vi "zero steering.vi"(9 "Power (100)":i8=100, 11 "NXT":T1={"error"={"status"=FALSE, "code"=0, "source"=""}, "address"="", "NXT #"=-1, "Show Error"=TRUE, "Connection"=4} {"Connection" items=["USB", "Bluetooth", "USB then Bluetooth", "Last Connection", "Preference"]}) -> (3 "NXT":T1={"error"={"status"=FALSE, "code"=0, "source"=""}, "address"="", "NXT #"=-1, "Show Error"=TRUE, "Connection"=4} {"Connection" items=["USB", "Bluetooth", "USB then Bluetooth", "Last Connection", "Preference"]})   [LabVIEW 2009]
uses:
  <vilib>/NXT/Subs/LVHSConnector.ctl
  <vilib>/NXT/Subs/MotorOutput.ctl
  <vilib>/NXT/Dual Mode Library/Motors/ResetMotor.vi
  <vilib>/NXT/Dual Mode Library/Motors/MotorBrake.vi
  <vilib>/NXT/Dual Mode Library/Motors/MotorOn.vi
  <vilib>/NXT/Dual Mode Library/Motors/Rotation.vi
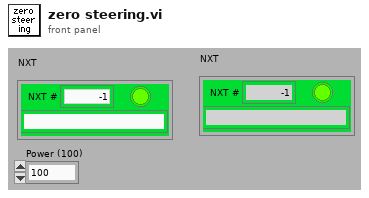
[diagram p1: front panel]
types:
  T1 = typedef "LVHSConnector.ctl" = cluster{"error":errorcluster, "address":string, "NXT #":i32, "Show Error":bool, "Connection":u16}
  T2 = typedef "MotorOutput.ctl" = u8
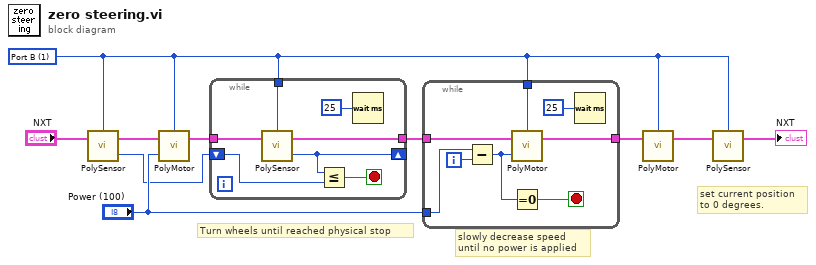
[diagram p0: block diagram]
diagram:
  w3 = T2 1 items=["Port A", "Port B", "Port C", "All Ports"] ("Output Port (All Ports)")
  # "Turn wheels until reached physical stop"
  # "set current position\nto 0 degrees."
  # "slowly decrease speed\nuntil no power is applied"
  n1 = call-poly <vilib>:"PolySensor.vi"("NXT"="NXT", "Port (Port A)"=w3) -> ("Rotation"=w1:i32, "NXT"=w4:T1)  [unwired: 1 in]
  n2 = call-poly <vilib>:"PolyMotor.vi"("Power (75)"="Power (100)", "NXT"=w4, "Output Port (All Ports)"=w3) -> ("NXT"=w2:T1)  [unwired: 1 in]
  n3 = while {
    tunnel: w2 -> [w16]
    tunnel: w3 -> [w17]
    tunnel: [w15] -> w6
    shift-right: [w13] -> _
    shift-left: w1 -> [w12]
    stop <- w11 stop-if-true
    n4 = call-poly <vilib>:"PolySensor.vi"("NXT"=w16, "Port (Port A)"=w17) -> ("Rotation"=w13:i32, "NXT"=w15:T1)  [unwired: 1 in]
    n5 = Less Or Equal?(x=w13, y=w12) -> (x <= y?=w11:bool)
    n6 = Wait (ms)(milliseconds to wait=u32 25) -> ()  [unwired: 1 out]
  }
  n7 = while {
    tunnel: w6 -> [w25]
    tunnel: [w19] -> w10
    tunnel: w3 -> [w21]
    tunnel: "Power (100)" -> [w20]
    i -> [w24]
    stop <- w22 stop-if-true
    n8 = Subtract(x=w20, y=w24) -> (x-y=w23:i32)
    n9 = call-poly <vilib>:"PolyMotor.vi"("Power (75)"=w23, "NXT"=w25, "Output Port (All Ports)"=w21) -> ("NXT"=w19:T1)  [unwired: 1 in]
    n10 = Equal To 0?(x=w23) -> (x = 0?=w22:bool)
    n11 = Wait (ms)(milliseconds to wait=u32 25) -> ()  [unwired: 1 out]
  }
  n12 = call-poly <vilib>:"PolyMotor.vi"("NXT"=w10, "Port (All Ports)"=w3) -> ("NXT"=w9:T1)  [unwired: 2 in]
  n13 = call-poly <vilib>:"PolySensor.vi"("NXT"=w9, "Port (All Ports)"=w3) -> ("NXT"=→"NXT":T1)  [unwired: 2 in]
